vi "WLAN_FrameBuild.vi"(8 "error in (no error)":errorcluster, 10 "Modulation parameter":T1, 11 "data in":i8[](array[numeric]) caption="input bit stream") -> (0 "error out":errorcluster, 1 "symbols":cdb[](array[numeric]), 2 "output bit stream 3":i8[](array[numeric]) caption="output bit stream", 3 "output array":cdb[](array[numeric]))   [LabVIEW 2018]
panel:
  out "size(s) 3":i32
  out "size(s) 2":i32
  out "size(s)":i32
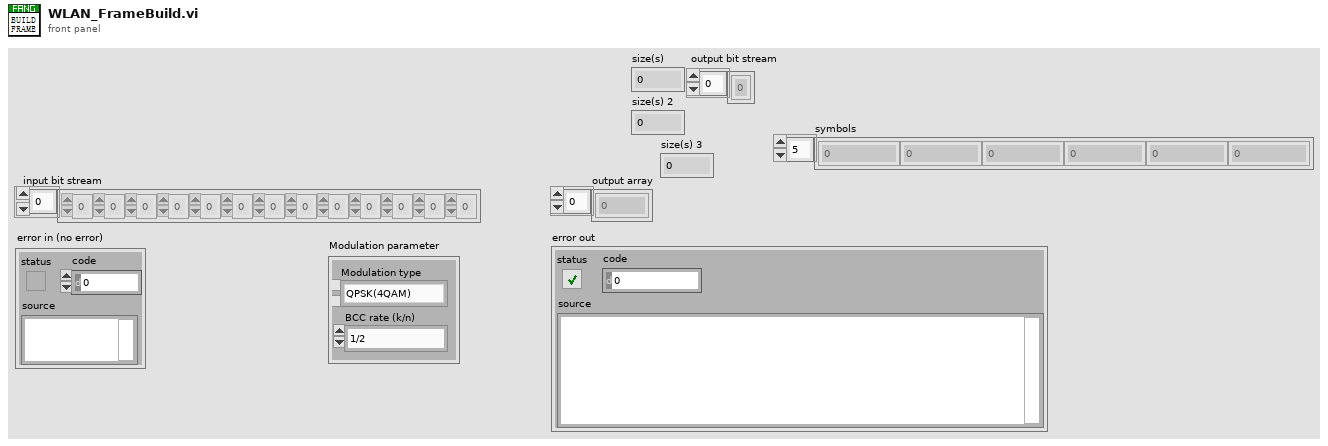
[diagram p1: front panel]
types:
  T1 = cluster{"Modulation type":enum16{"QPSK(4QAM)", "64QAM", "16QAM", "BPSK"}, "BCC rate (k/n)":enum16{"1/2", "2/3", "3/4"}}
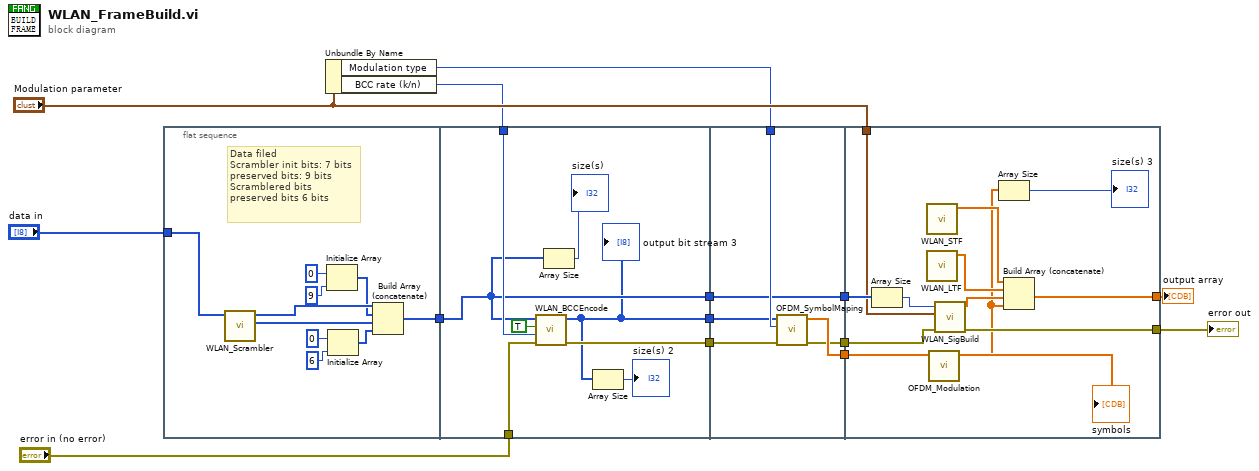
[diagram p0: block diagram]
diagram:
  n1 = flat-sequence {
    tunnel: "data in" -> [w24]
    tunnel: [w23] -> w13
    tunnel: w13 -> [w28]
    tunnel: "error in (no error)" -> [w31]
    tunnel: [w30] -> w11
    tunnel: [w26] -> w10
    tunnel: w7 -> [w29]
    tunnel: [w28] -> w2
    tunnel: w11 -> [w37]
    tunnel: w10 -> [w36]
    tunnel: w8 -> [w38]
    tunnel: [w35] -> w6
    tunnel: [w34] -> w5
    tunnel: w2 -> [w33]
    tunnel: [w33] -> w1
    tunnel: "Modulation parameter" -> [w48]
    tunnel: w6 -> [w47]
    tunnel: w5 -> [w44]
    tunnel: [w43] -> w4
    tunnel: [w40] -> w3
    tunnel: w1 -> [w50]
    frame #0 {
      # "Data filed\nScrambler init bits: 7 bits\npreserved bits: 9 bits\nScramblered bits\npreserved bits 6 bits"
      n2 = call "WLAN_Scrambler.vi"("input bit stream"=w24) -> ("scrambled bits"=w18:i8[], "scrambler initial bit"=w22:i8[])  [unwired: 9 in]
      n3 = Initialize Array(i8 0 ("element"), 9 ("dimension size")) -> (w21:i8[])
      n4 = Initialize Array(i8 0 ("element"), 6 ("dimension size")) -> (w15:i8[])
      n5 = Build Array (concatenate)(w22, w21, w18, w15) -> (w23:i8[])
    }
    frame #1 {
      n6 = call "WLAN_BCCEncode.vi"("error in (no error)"=w31, "BCC rate (k/n)"=w29, "need add zeros?"=TRUE, "input bit stream"=w28) -> ("error out"=w30:errorcluster, "output bit stream 3"=w26:i8[])  [unwired: 6 in]
      "output bit stream 3" <- w26
      n7 = Array Size(array=w28) -> (size(s)=→"size(s)":i32)
      n8 = Array Size(array=w26) -> (size(s)=→"size(s) 2":i32)
    }
    frame #2 {
      n9 = call "OFDM_SymbolMaping.vi"("error in (no error)"=w37, "Modulation type"=w38, "input bit stream"=w36) -> ("error out"=w34:errorcluster, "symbols"=w35:cdb[])  [unwired: 7 in]
    }
    frame #3 {
      n10 = Array Size(array=w50) -> (size(s)=w49:i32)
      n11 = call "WLAN_STF.vi"() -> ("STF"=w45:cdb[])  [unwired: 11 in]
      n12 = call "WLAN_LTF.vi"() -> ("LTF"=w46:cdb[])  [unwired: 11 in]
      n13 = call "OFDM_Modulation.vi"("Input sequence"=w47) -> ("Output sequence"=w39:cdb[])  [unwired: 10 in]
      n14 = call "WLAN_SigBuild.vi"("Data bit length"=w49, "Modulation parameter"=w48, "error in (no error)"=w44) -> ("symbols"=w42:cdb[], "error out"=w43:errorcluster)  [unwired: 6 in]
      n15 = Array Size(array=w39) -> (size(s)=→"size(s) 3":i32)
      n16 = Build Array (concatenate)(w45, w46, w42, w39) -> (w40:cdb[])
      "symbols" <- w47
    }
  }
  n17 = Unbundle By Name("Modulation parameter") -> ("Modulation type"=w8:enum16{"QPSK(4QAM)", "64QAM", "16QAM", "BPSK"}, "BCC rate (k/n)"=w7:enum16{"1/2", "2/3", "3/4"})
  "output array" <- w3
  "error out" <- w4
